vi "Has Focus Event_ACAF.vi"(8 "error in (no error)":errorcluster, 11 "Control Ref":refnum<vi>) -> (0 "error out":errorcluster, 3 "Key Focus UE":refnum<user-event>)   [LabVIEW 2023]
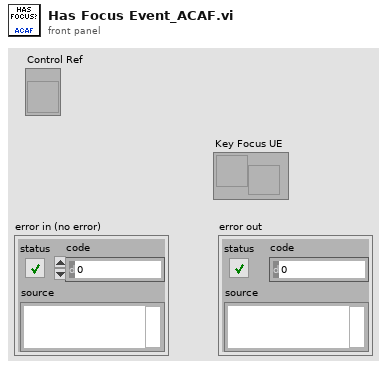
[diagram p1: front panel]
types:
  T1 = cluster{"Control Ref":refnum<vi>, "Has focus?":bool}
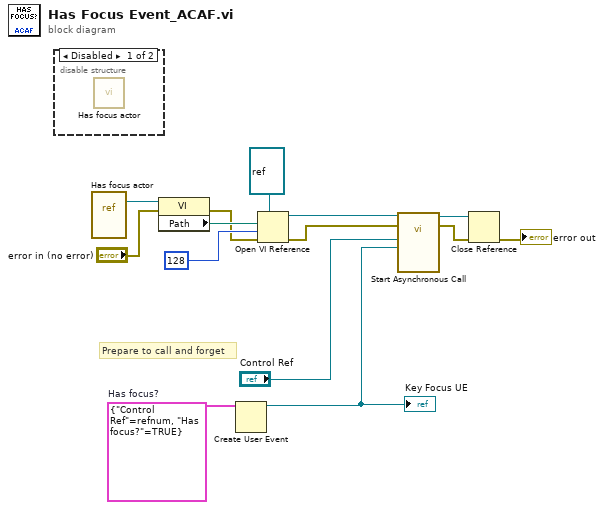
[diagram p0: block diagram]
diagram:
  w3 = T1 {"Control Ref"=refnum, "Has focus?"=TRUE}  # Has focus?
  # "Prepare to call and forget"
  n1 = disable-structure shown="Disabled" {
    frame Disabled {
      n2 = call "Has focus actor.vi"() -> ()  [unwired: 12 in]
    }
    frame Enabled {
    }
  }
  n3 = vi-ref "Has focus actor.vi"() -> (w14:refnum<vi>)
  n4 = property class="VI"(reference=w14, error in="error in (no error)") -> (error out=w4:errorcluster, "Path"=w10:path)  [unwired: 1 out]
  n5 = Create User Event(user event datatype=w3) -> (user event=w2:refnum<user-event>)  [unwired: 1 in, 1 out]
  "Key Focus UE" <- w2
  n6 = Open VI Reference(type specifier VI Refnum (for type only)=refnum<vi> refnum, vi path=w10, options=128, error in (no error)=w4) -> (vi reference=w5:refnum<vi>, error out=w9:errorcluster)  [unwired: 2 in]
  n7 = call-by-ref "Start Asynchronous Call"(reference=w5, error in=w9, "user event in"=w2, "Control Ref"="Control Ref") -> (reference out=w8:refnum<vi>, error out=w7:errorcluster)  [unwired: 10 in]
  n8 = Close Reference(reference=w8, error in (no error)=w7) -> (error out=→"error out":errorcluster)
